vi "WPI_RobotDriveOpen6MotorWithSPARK.vi"(0 "Rear Left Motor":T1, 1 "Rear Right Motor":T1, 2 "Front Right Motor":T1, 3 "Front Left Motor":T1, 4 "Mid Left Motor":T1, 5 "error in (no error)":errorcluster, 6 "Mid Right Motor":T1, 8 "Left Motors Inverted":bool, 10 "Right Motors Inverted":bool) -> (14 "RobotDriveDevRef":T2={"DevStatus"={"status"=FALSE, "code"=0, "source"=""}, "Motors[]"=[], "Square Inputs"=FALSE, "Max Output"=1.0}, 19 "error out":errorcluster)   [LabVIEW 2016, in "Drive System.lvlib"]
doc: "Opens a reference to the robot drive for a four-motor robot using CAN Jaguar motor controllers.\n\nThe CAN Jaguars are opened in Percent VBus mode. \n\nThis software is licensed. Open the labview\\readme\\WPI Robotics Library Open Source License.txt file for more information."
uses:
  <vilib>/Rock Robotics/SystemInterfaces/DIO/FPGA_DIOPWMChannel.ctl
  <vilib>/Rock Robotics/WPI/RobotDrive/WPI_RobotDriveDevRef.ctl
  <vilib>/Rock Robotics/WPI/MotorControl/WPI_MotorControlDeviceRef.ctl
  <vilib>/Rock Robotics/WPI/MotorControl/WPI_MotorControlType.ctl
  <vilib>/Rock Robotics/WPI/PWM/WPI_PWMDeadband.ctl
  <vilib>/Rock Robotics/WPI/SafetyOutput/WPI_SafetyOutputConfigMenu.ctl
  <vilib>/Rock Robotics/WPI/MotorControl/WPI_MotorControlOpen SPARK.vi
  SubSystems/Drive/Drive System.lvlib
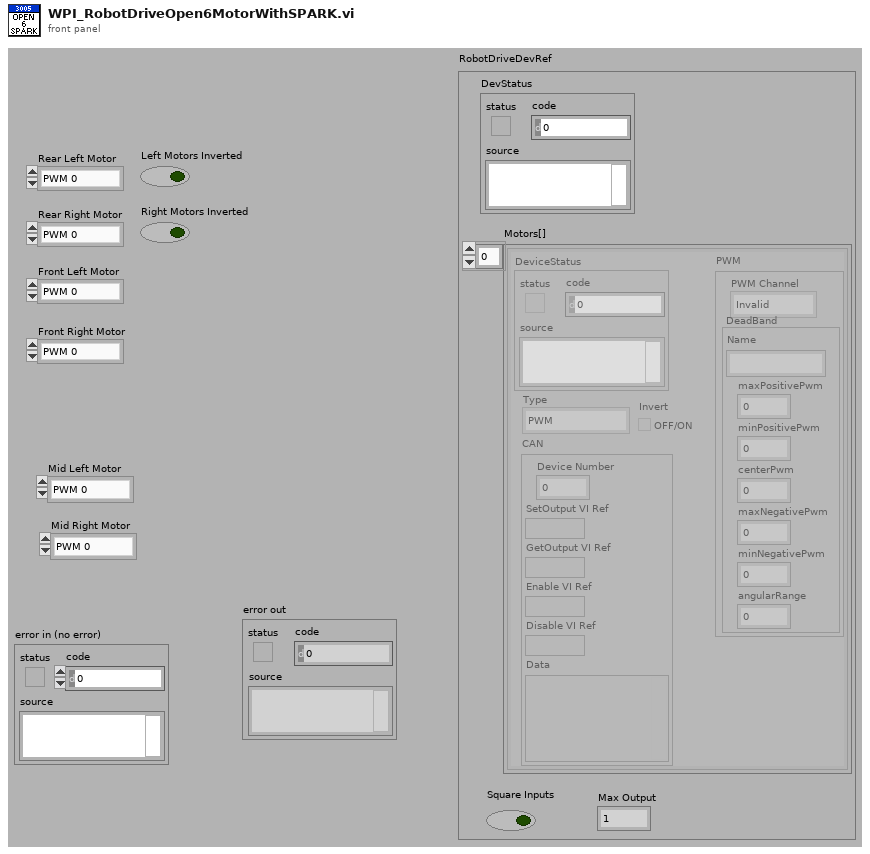
[diagram p1: front panel]
types:
  T1 = typedef "FPGA_DIOPWMChannel.ctl" = enum8{"PWM 0", "PWM 1", "PWM 2", "PWM 3", "PWM 4", "PWM 5", "PWM 6", "PWM 7", "PWM 8", "PWM 9", "PWM MXP 0", "PWM MXP 1", "PWM MXP 2", "PWM MXP 3", "PWM MXP 4", "PWM MXP 5", "PWM MXP 6", "PWM MXP 7", "PWM MXP 8", "PWM MXP 9", "Invalid"}
  T2 = typedef "WPI_RobotDriveDevRef.ctl" = cluster{"DevStatus":errorcluster, "Motors[]":T3[], "Square Inputs":bool, "Max Output":dbl}
  T3 = typedef "WPI_MotorControlDeviceRef.ctl" = cluster{"DeviceStatus":errorcluster, "Type":T4, "PWM":cluster{"PWM Channel":T1, "DeadBand":T5}, "CAN":cluster{"Device Number":u8, "SetOutput VI Ref":variant, "GetOutput VI Ref":variant, "Enable VI Ref":variant, "Disable VI Ref":variant, "Data":variant}, "Invert":bool}
  T4 = typedef "WPI_MotorControlType.ctl" = enum16{"PWM", "CAN"}
  T5 = typedef "WPI_PWMDeadband.ctl" = cluster{"Name":string, "maxPositivePwm":i32, "minPositivePwm":i32, "centerPwm":i32, "maxNegativePwm":i32, "minNegativePwm":i32, "angularRange":u16}
  T6 = typedef "WPI_SafetyOutputConfigMenu.ctl" = enum16{"Enable", "Disable"}
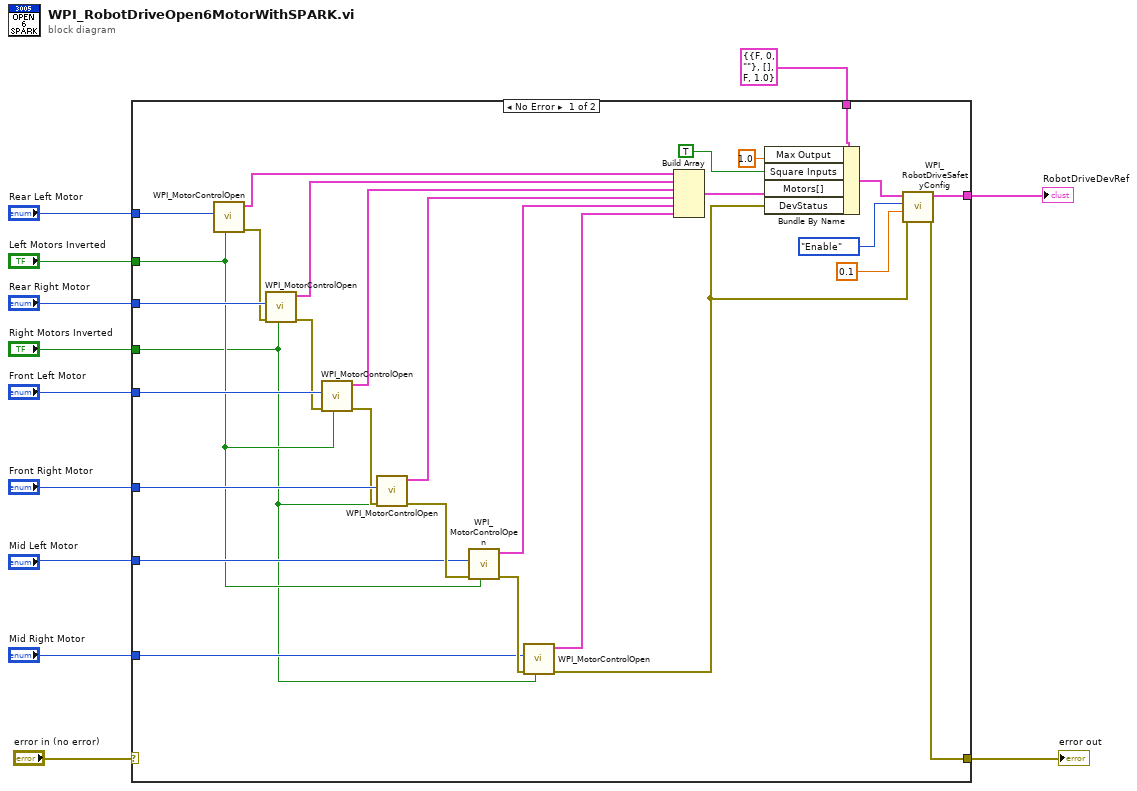
[diagram p0: block diagram]
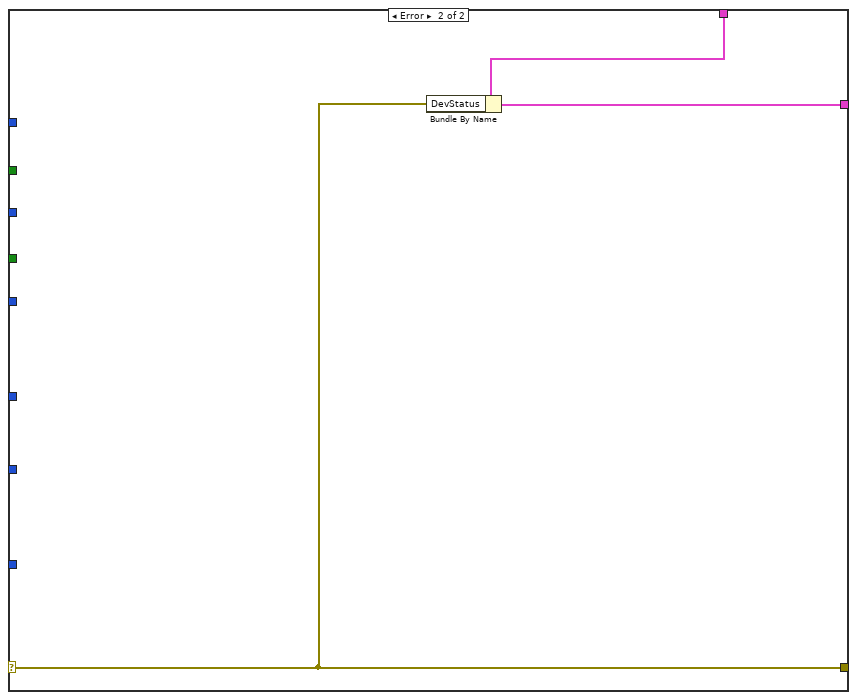
[diagram p2: hidden frame]
diagram:
  n1 = case shown="No Error" "error in (no error)" {
    selector: "error in (no error)" -> [_ w42]
    tunnel: [w24 w43] -> w12
    tunnel: T2 {"DevStatus"={"status"=FALSE, "code"=0, "source"=""}, "Motors[]"=[], "Square Inputs"=FALSE, "Max Output"=1.0} ("RobotDriveDevRef") -> [w41 w44]
    tunnel: "Rear Left Motor" -> [w39 _]
    tunnel: "Front Right Motor" -> [w36 _]
    tunnel: "Front Left Motor" -> [w37 _]
    tunnel: "Rear Right Motor" -> [w38 _]
    tunnel: "Left Motors Inverted" -> [w14 _]
    tunnel: "Right Motors Inverted" -> [w13 _]
    tunnel: [w25 w42] -> w3
    tunnel: "Mid Left Motor" -> [w16 _]
    tunnel: "Mid Right Motor" -> [w15 _]
    frame No Error {
      n2 = call-poly <vilib>:"WPI_MotorControlOpen.vi"("Invert"=w14, "PWM Channel"=w39) -> ("error out"=w29:errorcluster, "MotorControlDeviceRef"=w35:T3)  [unwired: 3 in, 5 out]
      n3 = call-poly <vilib>:"WPI_MotorControlOpen.vi"("Invert"=w13, "error in (no error)"=w29, "PWM Channel"=w38) -> ("error out"=w30:errorcluster, "MotorControlDeviceRef"=w34:T3)  [unwired: 2 in, 5 out]
      n4 = call-poly <vilib>:"WPI_MotorControlOpen.vi"("Invert"=w14, "error in (no error)"=w30, "PWM Channel"=w37) -> ("error out"=w31:errorcluster, "MotorControlDeviceRef"=w33:T3)  [unwired: 2 in, 5 out]
      n5 = call-poly <vilib>:"WPI_MotorControlOpen.vi"("Invert"=w13, "error in (no error)"=w31, "PWM Channel"=w36) -> ("error out"=w20:errorcluster, "MotorControlDeviceRef"=w32:T3)  [unwired: 2 in, 5 out]
      n6 = call-poly <vilib>:"WPI_MotorControlOpen.vi"("Invert"=w14, "error in (no error)"=w20, "PWM Channel"=w16) -> ("error out"=w21:errorcluster, "MotorControlDeviceRef"=w19:T3)  [unwired: 2 in, 5 out]
      n7 = call-poly <vilib>:"WPI_MotorControlOpen.vi"("Invert"=w13, "error in (no error)"=w21, "PWM Channel"=w15) -> ("error out"=w17:errorcluster, "MotorControlDeviceRef"=w18:T3)  [unwired: 2 in, 5 out]
      n8 = Build Array(w35, w34, w33, w32, w19, w18) -> (w28:T3[])
      n9 = Bundle By Name(cluster=w41, "Max Output"=1.0, "Square Inputs"=TRUE ("DestroyPWM?"), "Motors[]"=w28, "DevStatus"=w17) -> (w26:T2)
      n10 = call <vilib>:"WPI_RobotDriveSafetyConfig.vi"("error in (no error)"=w17, "timeout (s)"=0.1, "mode"=WPI_SafetyOutputConfigMenu."Enable", "RobotDriveDevRef"=w26) -> ("error out"=w25:errorcluster, "RobotDriveDevRef"=w24:T2)  [unwired: 6 out]
    }
    frame Error {
      n11 = Bundle By Name(cluster=w44, "DevStatus"=w42) -> (w43:T2)
    }
  }
  "RobotDriveDevRef" <- w12
  "error out" <- w3
